vi "obtain_resources.vi"(8 "error in (no error)":errorcluster) -> (0 "error out":errorcluster, 3 "LabJackRes":T1)   [LabVIEW 2025, in "LabJackEKG.lvlib"]
uses:
  Typedefs/LabJackGlobalResources.ctl
  Typedefs/LabJackQueues.ctl
  LabJackEKG.lvlib
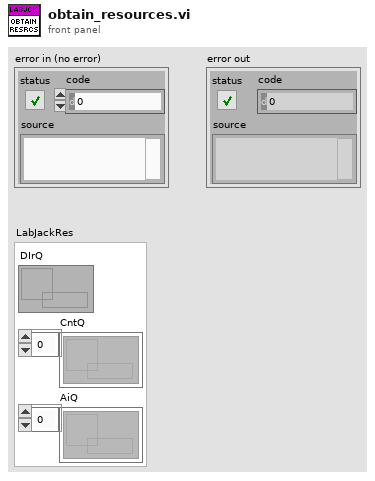
[diagram p1: front panel]
types:
  T1 = typedef "LabJackGlobalResources.ctl" = cluster{"DIrQ":refnum<queue>, "CntQ":refnum<queue>[], "AiQ":refnum<queue>[]}
  T2 = typedef "LabJackEKG.lvlib/LabJackQueues.ctl" = cluster{"DIrQ":refnum<queue>, "CntQ":refnum<queue>[], "AiQ":refnum<queue>[]}
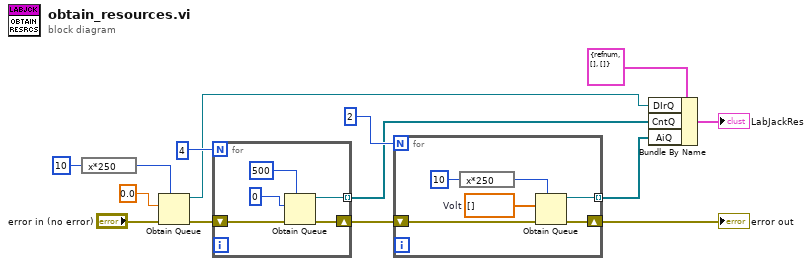
[diagram p0: block diagram]
diagram:
  n1 = expression code="x*250"(10 ("max queue size (-1, unlimited)")) -> (w1:i32)
  n2 = Obtain Queue(max queue size (-1, unlimited)=w1, element data type=0.0, error in (no error)="error in (no error)") -> (queue out=w5:refnum<queue>, error out=w10:errorcluster)  [unwired: 2 in, 1 out]
  n3 = for {
    N: 4 -> [_]
    tunnel: [w17] -> w4 mode=indexing
    shift-right: [w19] -> w9
    shift-left: w10 -> [w15]
    n4 = Obtain Queue(max queue size (-1, unlimited)=500, element data type=i64 0, error in (no error)=w15) -> (queue out=w17:refnum<queue>, error out=w19:errorcluster)  [unwired: 2 in, 1 out]
  }
  n5 = for {
    N: 2 -> [_]
    tunnel: [w24] -> w3 mode=indexing
    shift-right: [w21] -> w8
    shift-left: w9 -> [w20]
    w25 = dbl[] []  # Volt
    n6 = expression code="x*250"(10 ("max queue size (-1, unlimited)")) -> (w22:i32)
    n7 = Obtain Queue(max queue size (-1, unlimited)=w22, element data type=w25, error in (no error)=w20) -> (queue out=w24:refnum<queue>, error out=w21:errorcluster)  [unwired: 2 in, 1 out]
  }
  "error out" <- w8
  n8 = Bundle By Name(cluster=T2 {"DIrQ"=refnum, "CntQ"=[], "AiQ"=[]} ("Queues"), "DIrQ"=w5, "CntQ"=w4, "AiQ"=w3) -> (→"LabJackRes":T2)
